vi "niFPGA Threshold Crossing Logic.vi"(5 "reset":bool, 6 "le low ref":bool, 7 "ge high ref":bool, 8 "state in":T1={"level"=[FALSE, FALSE, FALSE, FALSE, FALSE, FALSE], "rising?"=FALSE, "hi hyst met?"=FALSE, "lo hyst met?"=FALSE, "gt threshold"=FALSE, "lt threshold"=FALSE}, 9 "direction":u8(ring) items=["falling", "rising"], 10 "lt threshold":bool, 11 "gt threshold":bool) -> (0 "state out":T1, 3 "crossing":bool)   [LabVIEW 2017]
uses:
  <vilib>/rvi/Analysis/utilities/niFPGA Threshold Crossing State.ctl
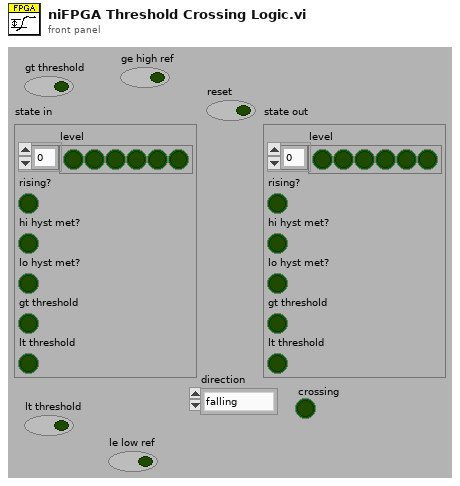
[diagram p1: front panel]
types:
  T1 = typedef "niFPGA Threshold Crossing State.ctl" = cluster{"level":bool[], "rising?":bool, "hi hyst met?":bool, "lo hyst met?":bool, "gt threshold":bool, "lt threshold":bool}
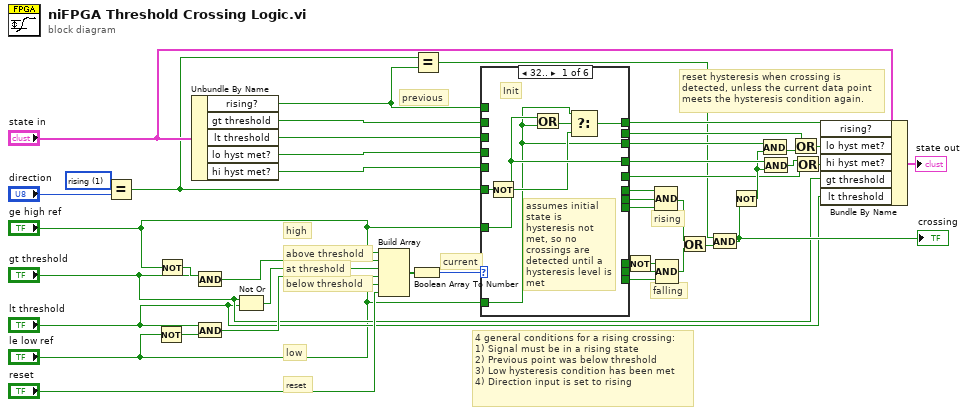
[diagram p0: block diagram]
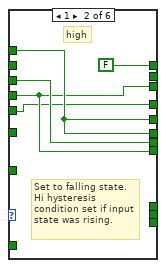
[diagram p2: hidden frame]
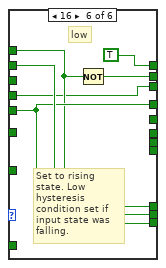
[diagram p6: hidden frame]
diagram:
  w28 = u8 1 items=["falling", "rising"] ("direction")
  # "reset"
  # "low"
  # "below threshold"
  # "at threshold"
  # "above threshold"
  # "high"
  # "rising"
  # "falling"
  # "reset hysteresis when crossing is detected, unless the current data point meets the hysteresis condition again."
  # "4 general conditions for a rising crossing:\n1) Signal must be in a rising state\n2) Previous point was below threshold\n3) Low hysteresis condition has been met\n4) Direction input is set to rising"
  # "current"
  # "previous"
  n1 = Equal?(x=w28, y="direction") -> (x = y?=w5:bool)
  n2 = Not(x="le low ref") -> (.not. x?=w43:bool)
  n3 = Not(x="ge high ref") -> (.not. x?=w44:bool)
  n4 = Unbundle By Name("state in") -> ("rising?"=w29:bool, "gt threshold"=w34:bool, "lt threshold"=w33:bool, "lo hyst met?"=w30:bool, "hi hyst met?"=w32:bool)
  n5 = And(x=w44, y="gt threshold") -> (x .and. y?=w42:bool)
  n6 = And(x="lt threshold", y=w43) -> (x .and. y?=w39:bool)
  n7 = Not Or(1:"lt threshold", 2:"gt threshold") -> (0:w41:bool)
  n8 = Build Array("ge high ref", w42, w41, w39, "le low ref", "reset") -> (w35:bool[])
  n9 = Boolean Array To Number(Boolean array=w35) -> (number=w40:u8)
  n10 = Equal?(x=w5, y=w29) -> (x = y?=w6:bool)
  n11 = case shown="32.." w40 {
    tunnel: [_ _ _ w64 w67 w71] -> w15
    tunnel: [w45 FALSE w58 w64 w67 TRUE] -> w36
    tunnel: w29 -> [_ w53 w58 w64 w67 w71]
    tunnel: w34 -> [_ _ _ w61 w66 w73]
    tunnel: w33 -> [_ w54 w57 w60 _ _]
    tunnel: w32 -> [_ w51 w59 w62 w65 w72]
    tunnel: [w49 w51 w59 w62 w65 w72] -> w27
    tunnel: [w46 w52 w56 w63 w68 w69] -> w26
    tunnel: w30 -> [_ w52 w56 w63 w68 w69]
    tunnel: "le low ref" -> [w46 _ _ _ _ _]
    tunnel: "ge high ref" -> [w49 _ _ _ _ _]
    tunnel: [_ _ _ _ _ w70] -> w21
    tunnel: [_ w53 _ _ _ _] -> w19
    tunnel: [_ w53 w58 w64 _ _] -> w14
    tunnel: [_ w54 w57 w63 _ _] -> w13
    tunnel: [_ w52 w56 w60 _ _] -> w12
    tunnel: [_ _ _ w62 w66 w73] -> w11
    tunnel: [_ _ _ w61 w65 w72] -> w10
    tunnel: w5 -> [w48 _ _ _ _ _]
    frame 32.. {
      # "assumes initial state is hysteresis not met, so no crossings are detected until a hysteresis level is met"
      # "Init"
      n12 = Not(x=w48) -> (.not. x?=w47:bool)
      n13 = Or(x=w49, y=w46) -> (x .or. y?=w50:bool)
      n14 = Select(t=w46, s=w50, f=w47) -> (s? t:f=w45:bool)
    }
    frame 1 {
      # "Set to falling state. Hi hysteresis condition set if input state was rising."
      # "high"
    }
    frame 2 {
      # "above threshold"
    }
    frame 4, Default {
      # "falling crossing"
      # "rising crossing"
      # "== threshold"
    }
    frame 8 {
      # "below threshold"
    }
    frame 16 {
      # "Set to rising state. Low hysteresis condition set if input state was falling."
      # "low"
      n15 = Not(x=w71) -> (.not. x?=w70:bool)
    }
  }
  n16 = Not(x=w15) -> (.not. x?=w9:bool)
  n17 = Compound Arithmetic op=AND(w14, w13, w12) -> (w17:bool)
  n18 = Compound Arithmetic op=AND(w9, w11, w10) -> (w18:bool)
  n19 = Or(x=w17, y=w18) -> (x .or. y?=w16:bool)
  n20 = And(x=w6, y=w16) -> (x .and. y?=w7:bool)
  "crossing" <- w7
  n21 = Not(x=w7) -> (.not. x?=w20:bool)
  n22 = And(x=w26, y=w20) -> (x .and. y?=w25:bool)
  n23 = And(x=w27, y=w20) -> (x .and. y?=w24:bool)
  n24 = Or(x=w21, y=w25) -> (x .or. y?=w22:bool)
  n25 = Or(x=w24, y=w19) -> (x .or. y?=w23:bool)
  n26 = Bundle By Name(cluster="state in", "rising?"=w36, "lo hyst met?"=w22, "hi hyst met?"=w23, "gt threshold"="gt threshold", "lt threshold"="lt threshold") -> (→"state out":T1)
